vi "ReceiveCapturedImage.vi"(8 "error in (no error)":errorcluster, 10 "JSON":string, 11 "TopLevel in":refnum<class "TopLevel.lvclass">) -> (0 "error out":errorcluster, 3 "TopLevel out":refnum<class "TopLevel.lvclass">)   [LabVIEW 2021, in "TopLevel.lvlib" / "TopLevel.lvclass"]
uses:
  TopLevel.lvclass
  TopLevel.lvclass/TopLevel.ctl
  Models/ImagesModel.ctl
  Typedef/ImageResults.ctl
  Models/InferenceDataModel.ctl
  AI Inference/Inference/Inference Messages/Process Msg/Process Msg.lvclass/Process Msg.ctl
  <vilib>/ActorFramework/Message Enqueuer/Message Enqueuer.lvclass/Message Enqueuer.ctl
  02442360-9df0-45be-85d0-8fe4040f395d.vi
  48e57916-1b3b-418a-ac96-857321cf0a90.vi
  <vilib>/ActorFramework/Message Enqueuer/Enqueue.vi
  AI Inference/Inference/Inference Messages/Process Msg/Process Msg.lvclass
  C:/Program Files (x86)/National Instruments/LabVIEW 2021/vi.lib/ActorFramework/Message/Message.lvclass
  <vilib>/JDP Science/JSONtext/JSON text to Variant.vi
  <vilib>/JDP Science/JSONtext/Variant to JSON Text.vi
  <vilib>/ActorFramework/Message Priority Queue/Priority Enqueue.vi
  <vilib>/JDP Science/JSONtext/LVClass Serializer/JSONtext LVClass Serializer.lvclass
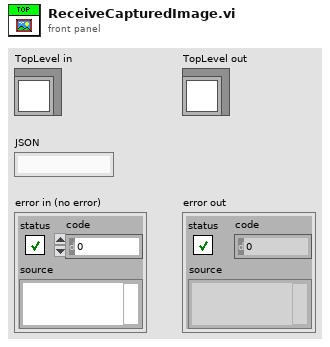
[diagram p1: front panel]
types:
  T1 = typedef "InferenceDataModel.ctl" = cluster{"guid":string, "images":string[]}
  T2 = cluster{"image":string, "pass":bool, "class":string}
  T3 = typedef "TopLevel.lvlib/TopLevel.lvclass/ImageResults.ctl" = cluster{"source":cluster{"image":string, "pass":bool, "class":string}, "rois":cluster{"image":string, "pass":bool, "class":string}[]}
  T4 = typedef "ImagesModel.ctl" = cluster{"guid":string, "images":cluster{"source":string, "rois":string[]}}
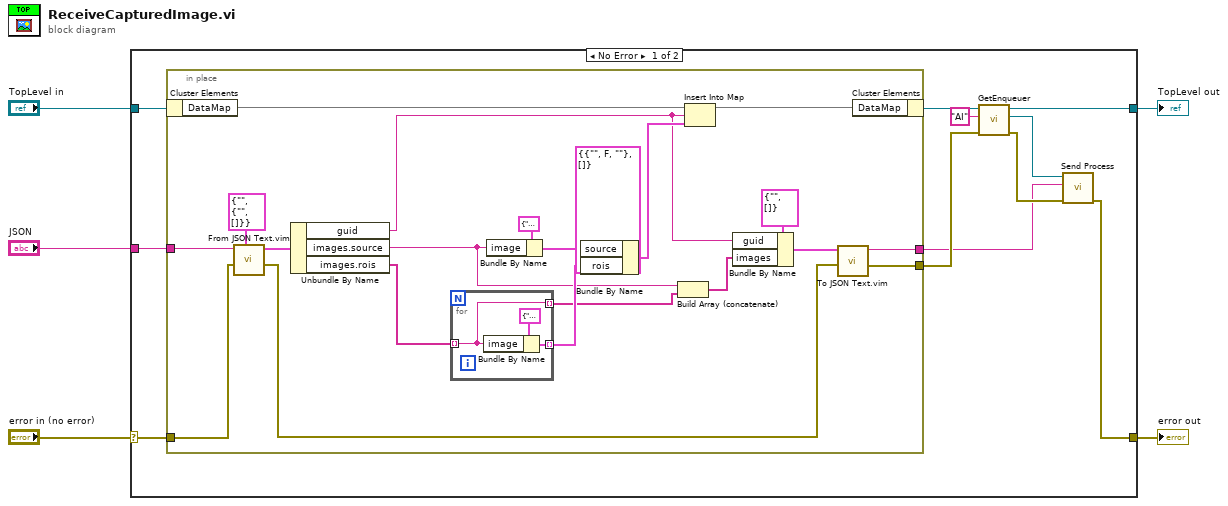
[diagram p0: block diagram]
diagram:
  n1 = case shown="No Error" "error in (no error)" {
    selector: "error in (no error)" -> [w15 w42]
    tunnel: [w8 w42] -> w4
    tunnel: [w10 w41] -> w2
    tunnel: "TopLevel in" -> [w14 w41]
    tunnel: "JSON" -> [w16 _]
    frame No Error {
      n2 = in-place {
        in-place-border: w16 -> [w35]
        in-place-border: w15 -> [w34]
        in-place-border: [w18] -> w7
        in-place-border: [w17] -> w6
        n3 = in-place-cluster #1(w14) -> ("DataMap"=w37:map{string, T3})
        n4 = call "From JSON Text.vim"("Data Type and Default Value"=T4 {"guid"="", "images"={"source"="", "rois"=[]}} ("Cluster"), "error in (no error)"=w34, "JSON"=w35) -> ("error out"=w19:errorcluster, "Data out"=w32:T4)  [unwired: 7 in]
        n5 = Unbundle By Name(w32) -> ("guid"=w24:string, "images.source"=w23:string, "images.rois"=w28:string[])
        n6 = for {
          tunnel: w28 -> [w38] mode=indexing
          tunnel: [w39] -> w27 mode=indexing
          tunnel: [w38] -> w22 mode=indexing
          n7 = Bundle By Name(cluster=T2 {"image"="", "pass"=FALSE, "class"=""} ("source"), "image"=w38) -> (w39:T2)
        }
        n8 = Bundle By Name(cluster=T2 {"image"="", "pass"=FALSE, "class"=""} ("source"), "image"=w23) -> (w29:T2)
        n9 = Bundle By Name(cluster=T3 {"source"={"image"="", "pass"=FALSE, "class"=""}, "rois"=[]} ("value"), "source"=w29, "rois"=w27) -> (w26:T3)
        n10 = Build Array (concatenate)(w23, w22) -> (w21:string[])
        n11 = Insert Into Map(map in=w37, key=w24, value=w26) -> (map out=w36:map{string, T3})  [unwired: 2 out]
        n12 = Bundle By Name(cluster=T1 {"guid"="", "images"=[]} ("Data"), "guid"=w24, "images"=w21) -> (w20:T1)
        n13 = call "To JSON Text.vim"("error in (no error)"=w19, "Anything"=w20) -> ("error out"=w18:errorcluster, "<JSON>"=w17:string)  [unwired: 8 in]
        n14 = in-place-cluster #1("DataMap"=w36) -> (w13:refnum<class "TopLevel.lvclass">)
      }
      n15 = call "GetEnqueuer.vi"("error in (no error)"=w7, "Actor Name"="AI", "TopLevel in"=w13) -> ("error out"=w9:errorcluster, "Enqueuer"=w11:refnum<class "Message Enqueuer.lvclass">, "TopLevel out"=w10:refnum<class "TopLevel.lvclass">)  [unwired: 6 in]
      n16 = call "Send Process.vi"("error in (no error)"=w9, "Json Data"=w6, "Message Enqueuer"=w11) -> ("error out"=w8:errorcluster)  [unwired: 7 in, 1 out]
    }
    frame Error {
    }
  }
  "error out" <- w4
  "TopLevel out" <- w2
